vi "测试写设置.vi"() -> ()   [LabVIEW 2012, in "m_Lib.lvlib"]
uses:
  <userlib>/m_Lib/m_Lib.lvlib
  <userlib>/m_Lib/Setting/Demo/Data.ctl
panel:
  in  "簇":T1
  out "Error_Out":errorcluster
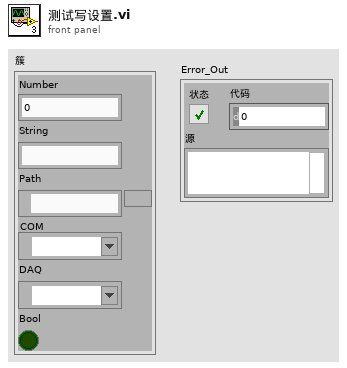
[diagram p1: front panel]
types:
  T1 = typedef "m_Lib.lvlib/Data.ctl" = cluster{"Number":u32, "String":string, "Path":path, "COM":refnum<visa-resource-name>, "DAQ":tag, "Bool":bool}
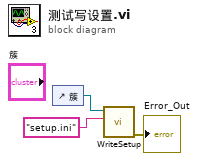
[diagram p0: block diagram]
diagram:
  n1 = control-ref of="簇"() -> (w1:refnum<vi>)
  n2 = call <userlib>:"WriteSetup.vi"("ConfigName"="setup.ini" ("名称或相对路径"), "Cluster_Quotes"=w1) -> ("Error_Out"=→"Error_Out":errorcluster)  [unwired: 8 in, 1 out]
